vi "is-valid.vi"(10 "ID":refnum<class "ID.lvclass">) -> (2 "is-valid?":bool)   [LabVIEW 2020, in "graph.lvlib" / "ID.lvclass"]
uses:
  ID.lvclass
  ID.lvclass/ID.ctl
  support/UUID/UUID.lvclass
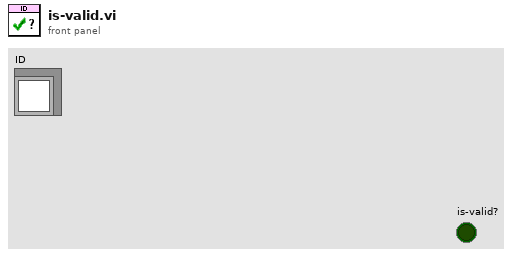
[diagram p1: front panel]
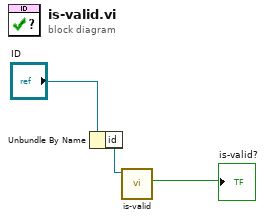
[diagram p0: block diagram]
diagram:
  n1 = Unbundle By Name("ID") -> ("id"=w2:refnum<class "UUID.lvclass">)
  n2 = call "is-valid.vi"("UUID in"=w2) -> ("is-valid?"=→"is-valid?":bool)  [unwired: 10 in]
